vi "Fetch VIPM Repos.vi"   [LabVIEW 2020]
uses:
  Libraries/Packages/VIPM/VIPM.lvlib
  Libraries/WSsupport/WSsupport.lvlib
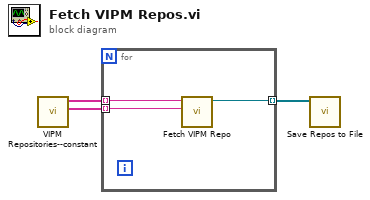
[diagram p0: block diagram]
diagram:
  n1 = call "VIPM Repositories--constant.vi"() -> ("Index Filenames"=w2:string[], "Repo URLs"=w3:string[])  [unwired: 10 in]
  n2 = for {
    tunnel: w3 -> [w6] mode=indexing
    tunnel: w2 -> [w5] mode=indexing
    tunnel: [w4] -> w1 mode=indexing
    n3 = call "Fetch VIPM Repo.vi"("Index filename"=w5, "Repo URL"=w6) -> ("Repo"=w4:refnum<class "Repo.lvclass">)  [unwired: 8 in, 1 out]
  }
  n4 = call "Save Repos to File.vi"("Repos"=w1) -> ()  [unwired: 9 in, 2 out]
